vi "ep_Check Input Size Equals Three.vi"(8 "error in (no error)":errorcluster, 11 "# of channels":i32) -> (0 "error out":errorcluster)   [LabVIEW 2014, in "NI_EP_Motor Monitoring.lvlib"]
uses:
  <vilib>/addons/Electrical Power/Motor Monitoring/NI_EP_Motor Monitoring.lvlib
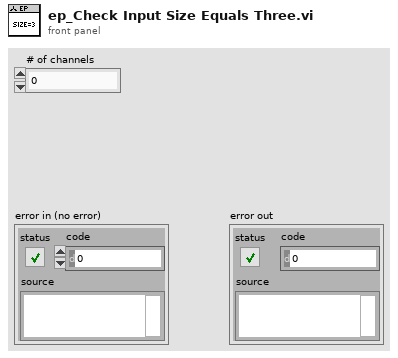
[diagram p1: front panel]
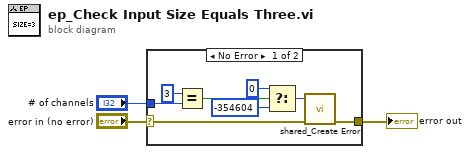
[diagram p0: block diagram]
diagram:
  n1 = case shown="No Error" "error in (no error)" {
    selector: "error in (no error)" -> [w9 w12]
    tunnel: "# of channels" -> [w11 _]
    tunnel: [w4 w12] -> w1
    frame No Error {
      n2 = Equal?(x=3, y=w11) -> (x = y?=w8:bool)
      n3 = Select(t=0 ("error code (0)"), s=w8, f=-354604 ("error code (0)")) -> (s? t:f=w7:i32)
      n4 = call <vilib>:"shared_Create Error.vi"("error in (no error)"=w9, "error code (0)"=w7) -> ("error out"=w4:errorcluster)  [unwired: 9 in]
    }
    frame Error {
    }
  }
  "error out" <- w1
